vi "Trace mMc.vi"(0 "Tr param":cluster{"T nr":i32, "T rt":i32, "T pos":dbl}={"T nr"=1, "T rt"=1, "T pos"=0.0} {"T rt" min=1 max=10000 step=1; "T nr" min=1 max=250 step=1}, 1 "Port":T1={"P type"=0, "reference"="", " Terminator "="\r\n", "Timeout"=300} {"Timeout" step=10; "P type" items=["none", "RS-232C"]}, 3 "error in (no error)":errorcluster, 4 "set/get":bool caption="set\n\n\nget", 5 "Controller #":string) -> (6 "# samples":i32, 7 "Tr ret":string, 9 "error out":errorcluster)   [LabVIEW 2011]
panel:
  # "Trace"
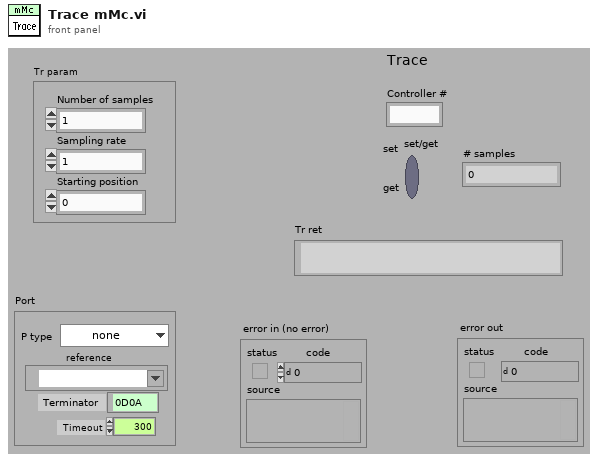
[diagram p1: front panel]
types:
  T1 = cluster{"P type":u16, "reference":refnum<visa-resource-name>, " Terminator ":string, "Timeout":i32}
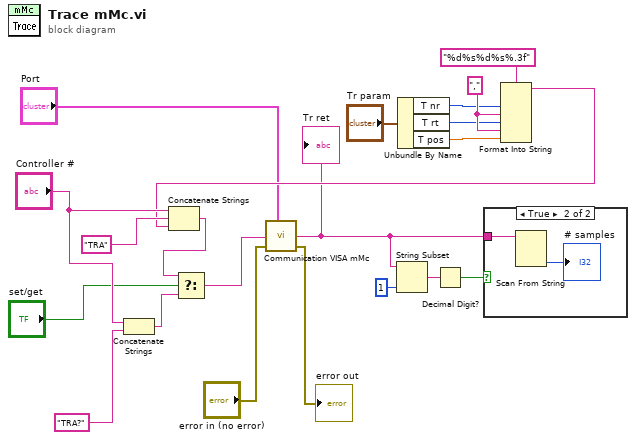
[diagram p0: block diagram]
diagram:
  w10 = ","
  n1 = Concatenate Strings("Controller #", "TRA?") -> (w21:string)
  n2 = Unbundle By Name("Tr param") -> ("T nr"=w7:i32, "T rt"=w6:i32, "T pos"=w5:dbl)
  n3 = Format Into String(format string="%d%s%d%s%.3f", w7, w10, w6, w10, w5) -> (resulting string=w12:string)  [unwired: 2 in, 1 out]
  n4 = Concatenate Strings("Controller #", "TRA", w12) -> (w19:string)
  n5 = Select(t=w19, s="set/get", f=w21) -> (s? t:f=w18:string)
  n6 = call "Communication VISA mMc.vi"("Port"="Port", "Command"=w18, "error in (no error)"="error in (no error)") -> ("Return"=w1:string, "error out"=→"error out":errorcluster)  [unwired: 3 in, 2 out]
  "Tr ret" <- w1
  n7 = String Subset(string=w1, length (rest)=1 ("length (rest)")) -> (substring=w3:string)  [unwired: 1 in]
  n8 = Decimal Digit?(1:w3) -> (0:w2:bool)
  n9 = case shown="True" w2 {
    tunnel: w1 -> [_ w22]
    frame False {
    }
    frame True {
      n10 = Scan From String(input string=w22) -> (output 1=→"# samples":i32)  [unwired: 4 in, 3 out]
    }
  }
